vi "Get Scaled BD to PictureBox.vi"(8 "错误输入（无错误）":errorcluster, 10 "图像参数":cluster{"图像深度":i32, "最大宽度":i32, "最大高度":i32}={"图像深度"=8, "最大宽度"=0, "最大高度"=0} {"图像深度" items=["1位、黑白"=1, "4位、16色"=4, "8位、256色"=8, "24位、真彩色"=24]}, 11 "VI Ref":refnum<vi>) -> (0 "错误输出":errorcluster, 3 "BD图像":picture)   [LabVIEW 2012, in "VIRef.lvlib"]
uses:
  VIRef.lvlib
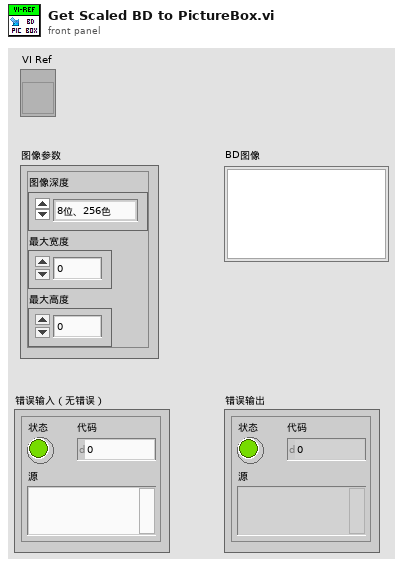
[diagram p1: front panel]
types:
  T1 = typedef "imagedata.ctl" = cluster{"image type":i32, "image depth":i32, "image":u8[], "mask":u8[], "colors":u32[], "Rectangle":cluster{"left":i16, "top":i16, "right":i16, "bottom":i16}}
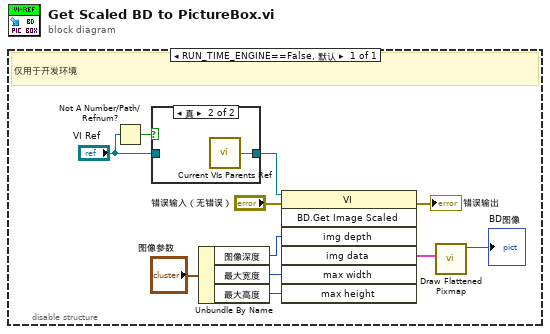
[diagram p0: block diagram]
diagram:
  n1 = disable-structure shown="RUN_TIME_ENGINE==False, 默认" {
    frame condition #0 (active) {
      # "仅用于开发环境"
      n2 = Not A Number/Path/Refnum?(number/path/refnum="VI Ref") -> (NaN/Path/Refnum?=w11:bool)
      n3 = case shown="真" w11 {
        tunnel: [w12 w13] -> w9
        tunnel: "VI Ref" -> [w12 _]
        frame False {
        }
        frame True {
          n4 = call "Current VIs Parents Ref.vi"() -> ("Calling VI's Reference"=w13:refnum<vi>)  [unwired: 2 in]
        }
      }
      n5 = Unbundle By Name("图像参数") -> ("图像深度"=w3:i32, "最大宽度"=w2:i32, "最大高度"=w1:i32)
      n6 = invoke class="VI" method="BD.Get Image Scaled"(reference=w9, error in="错误输入（无错误）", "img depth"=w3, "max width"=w2, "max height"=w1) -> (error out=→"错误输出":errorcluster, "img data"=w6:T1)  [unwired: 2 in, 5 out]
      n7 = call <vilib>:"Draw Flattened Pixmap.vi"("image data"=w6) -> ("new picture"=→"BD图像":picture)  [unwired: 8 in]
    }
  }
